vi "20T_CS_schleife.vi"   [LabVIEW 2016]
uses:
  Monitors/Utility/Monitor Communication/Gustav/20T_Control.ctl
  Global/Global Variables/global.vi
  Monitors/Utility/Monitor Communication/sub-vis/20T_Open_Queue.vi
  Monitors/Utility/Monitor Communication/sub-vis/20T_Queue_Commands.vi
  Instrument_Setup.vi
  Global/Global Variables/Data_Display_global.vi
types:
  T1 = typedef "20T_Control.ctl" = cluster{"Clamp":bool, "Switch Heater":bool, "Go to Zero":bool, "Go to Set":bool, "Go to Hold":bool, "Setpoint (T)":dbl, "Rate (T/min)":dbl, "Set Rate":bool}
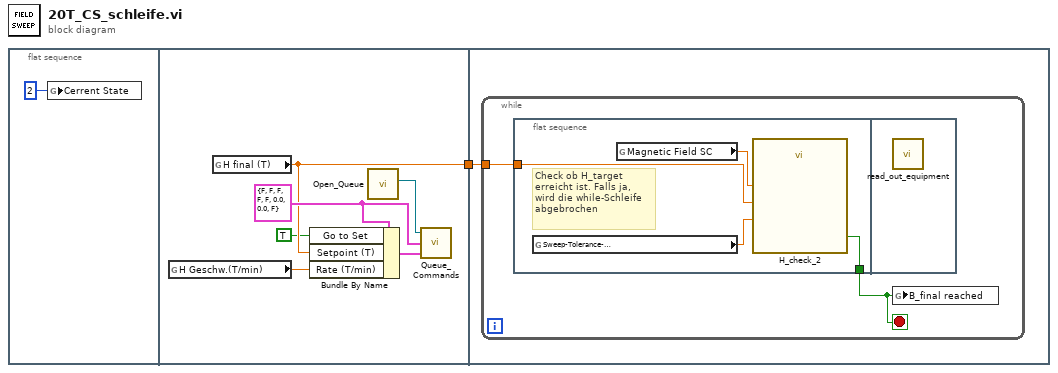
[diagram p0: block diagram]
diagram:
  n1 = flat-sequence {
    tunnel: [w5] -> w1
    tunnel: w1 -> [w9]
    frame #0 {
      n2 = global write "global.vi" "Cerrent State"(2) -> ()
    }
    frame #1 {
      w7 = T1 {"Clamp"=FALSE, "Switch Heater"=FALSE, "Go to Zero"=FALSE, "Go to Set"=FALSE, "Go to Hold"=FALSE, "Setpoint (T)"=0.0, "Rate (T/min)"=0.0, "Set Rate"=FALSE} ("Last Status")
      n3 = global read "global.vi" "H Geschw.(T/min)"() -> (w4:dbl)
      n4 = global read "global.vi" "H final (T)"() -> (w5:dbl)
      n5 = Bundle By Name(cluster=w7, "Go to Set"=TRUE, "Setpoint (T)"=w5, "Rate (T/min)"=w4) -> (w6:T1)
      n6 = call-poly "Open_Queue.vi"() -> ("queue out"=w8:refnum<queue>)  [unwired: 10 in, 1 out]
      n7 = call-poly "Queue_Commands.vi"("20 T Control"=w6, "Last Status"=w7, "20T Queue"=w8) -> ()  [unwired: 1 out]
    }
    frame #2 {
      n8 = while {
        tunnel: w9 -> [w10]
        stop <- w11 stop-if-true
        n9 = flat-sequence {
          tunnel: [w15] -> w11
          tunnel: w10 -> [w13]
          frame #0 {
            # "Check ob H_target\nerreicht ist. Falls ja,\nwird die while-Schleife\nabgebrochen"
            n10 = global read "Instrument_Setup.vi" "Sweep-Tolerance-\nMagnetic-Field"() -> (w14:dbl)
            n11 = global read "Data_Display_global.vi" "Magnetic Field SC"() -> (w12:dbl)
            n12 = call "H_check_2.vi"("Sweep\nTolerance %"=w14, "H_in"=w12, "H_target (K)"=w13) -> ("= H target"=w15:bool)  [unwired: 8 in]
          }
          frame #1 {
            n13 = call "read_out_equipment.vi"() -> ()  [unwired: 1 in]
          }
        }
        n14 = global write "Data_Display_global.vi" "B_final reached"(w11) -> ()
      }
    }
  }
